vi "w.vi"(8 "error in (no error)":errorcluster, 10 "ControlMouseUpMsg":refnum<class "ControlMouseUpMsg.lvclass">, 11 "TopButton In":refnum<class "TopButton.lvclass">) -> (0 "error out":errorcluster, 3 "TopButton Out":refnum<class "TopButton.lvclass">)   [LabVIEW 2017, in "TopButton.lvlib" / "TopButton.lvclass"]
doc: "<License>\nCopyright © 2017 Composed Systems, LLC | All rights reserved\nwww.composed.io\n\nAuthor: Ethan Stern <ethan.stern@composed.io>\n\nThis software is provided \"AS IS\" WITHOUT WARRANTIES, either express or implied, AND IS FOR EDUCATIONAL PURPOSES ONLY.\n</License>"
uses:
  <vilib>/gpm_packages/TestSystem/Views/TopButton/TopButton/TopButton.lvclass
  <vilib>/gpm_packages/@cs/mva-viewable/Source/ActorEvents/IEventAggregator Messages/ControlMouseUpMsg/ControlMouseUpMsg.lvclass
  <vilib>/gpm_packages/@cs/mva-viewable/Source/ActorEvents/IEventAggregator Messages/ControlMouseUpMsg/ControlMouseUpMsg.lvclass/ControlMouseUpMsg.ctl
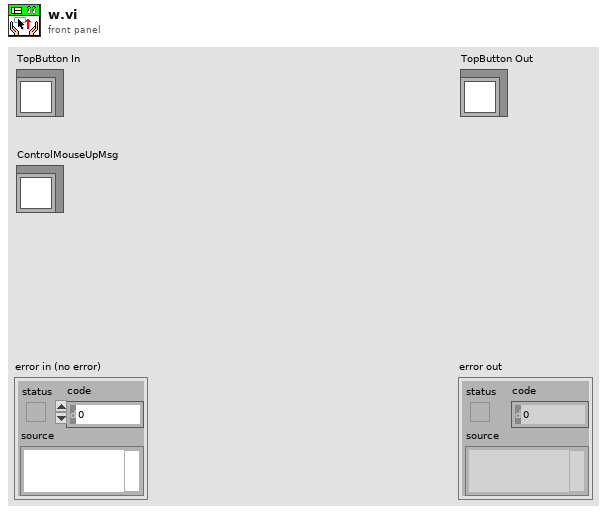
[diagram p1: front panel]
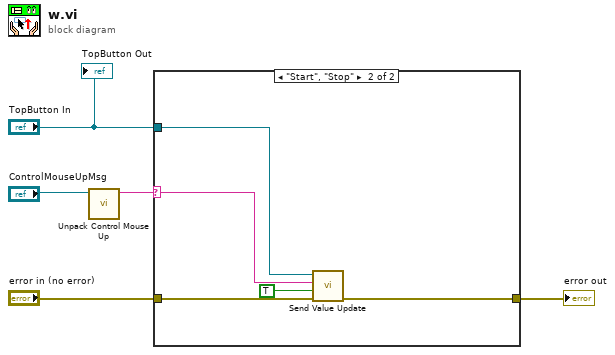
[diagram p0: block diagram]
diagram:
  n1 = call <vilib>:"Unpack Control Mouse Up.vi"("ControlMouseUpMsg"="ControlMouseUpMsg") -> ("Control Label"=w4:string)  [unwired: 4 in, 6 out]
  n2 = case shown="\"Start\", \"Stop\"" w4 {
    selector: w4 -> [_ w10]
    tunnel: "error in (no error)" -> [w6 w8]
    tunnel: "TopButton In" -> [_ w11]
    tunnel: [w6 w7] -> w2
    frame "False", Default {
    }
    frame "Start", "Stop" {
      n3 = call-dynamic "Send Value Update.vi"("error in (no error)"=w8, "Value"=TRUE, "Datum Name"=w10, "IViewable in"=w11) -> ("error out"=w7:errorcluster)  [unwired: 7 in]
    }
  }
  "error out" <- w2
  "TopButton Out" <- "TopButton In"
